vi "Month Load All Records.vi"(8 "error in (no error)":errorcluster, 10 "SQL Date":string, 11 "Database in":refnum<class "Database.lvclass">) -> (0 "error out":errorcluster, 2 "Statements":refnum<class "Statement.lvclass">[](array[class]), 3 "Database out":refnum<class "Database.lvclass">)   [LabVIEW 2018, in "Database.lvclass"]
uses:
  Database.lvclass
  Statement/Statement.lvclass
  Banking Statement/Banking Statement.lvclass
  C:/Users/jtipps/Documents/Filthy-Lucre-Budgetizer/source/support/classes/Statement/Statement.lvclass
  Credit Statement/Credit Statement.lvclass
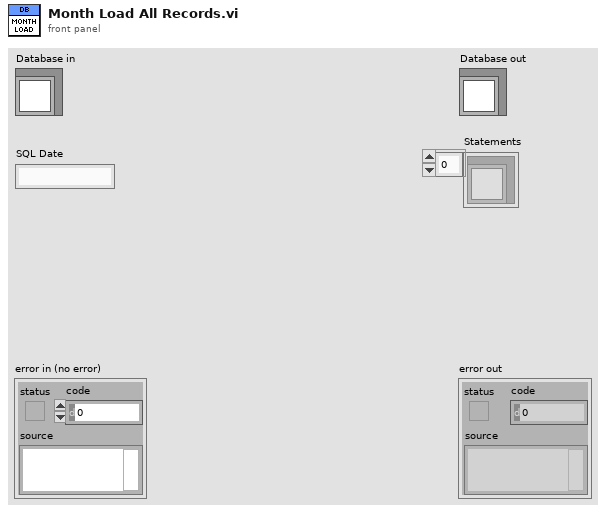
[diagram p1: front panel]
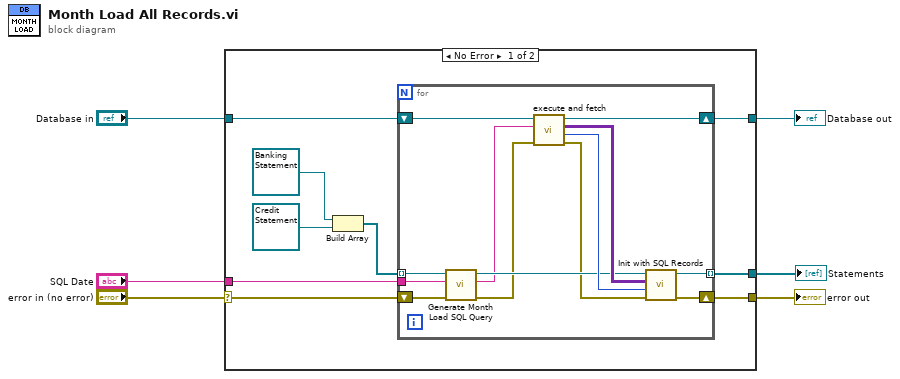
[diagram p0: block diagram]
diagram:
  n1 = case shown="No Error" "error in (no error)" {
    selector: "error in (no error)" -> [w12 w30]
    tunnel: [w13 w30] -> w3
    tunnel: [w14 w29] -> w6
    tunnel: "Database in" -> [w15 w29]
    tunnel: "SQL Date" -> [w10 _]
    tunnel: [w11 _] -> w1
    frame No Error {
      n2 = Build Array(refnum<class "Banking Statement.lvclass"> refnum ("Banking Statement.lvclass"), refnum<class "Credit Statement.lvclass"> refnum ("Credit Statement.lvclass")) -> (w9:refnum<class "Statement.lvclass">[])
      n3 = for {
        shift-right: [w27] -> w14
        shift-left: w15 -> [w28]
        shift-right: [w26] -> w13
        shift-left: w12 -> [w22]
        tunnel: [w25] -> w11 mode=indexing
        tunnel: w10 -> [w19]
        tunnel: w9 -> [w21] mode=indexing
        n4 = call-dynamic "Generate Month Load SQL Query.vi"("error in (no error)"=w22, "SQL Date"=w19, "Statement in"=w21) -> ("error out"=w17:errorcluster, "SQL Query"=w18:string, "Statement out"=w20:refnum<class "Statement.lvclass">)  [unwired: 6 in]
        n5 = call "execute and fetch.vi"("error in (no error)"=w17, "SQL query"=w18, "Database in"=w28) -> ("error out"=w16:errorcluster, "Num records"=w23:i32, "recordset data"=w24:variant[][], "Database out"=w27:refnum<class "Database.lvclass">)  [unwired: 5 in]
        n6 = call-dynamic "Init with SQL Records.vi"("error in (no error)"=w16, "Num records"=w23, "SQL Dataset"=w24, "Statement in"=w20) -> ("error out"=w26:errorcluster, "Statement out"=w25:refnum<class "Statement.lvclass">)  [unwired: 6 in]
      }
    }
    frame Error {
    }
  }
  "error out" <- w3
  "Database out" <- w6
  "Statements" <- w1
